vi "test - github 85 cannot write parameters into empty ini.vi"(8 "error in (no error)":errorcluster, 11 "TestCase in":refnum<class "csm-ini-variable-addon.lvclass">) -> (0 "error out":errorcluster, 3 "TestCase out":refnum<class "csm-ini-variable-addon.lvclass">)   [LabVIEW 2017, in "csm-ini-variable-addon.lvclass"]
uses:
  csm-ini-variable-addon.lvclass
  fd1f1403-f650-4147-a5d0-7fa8994ff20a.vi
  a890fef7-7f1d-42c9-b9db-12bb2b441289.vi
  25df91f5-a8e9-4b30-a15a-ad417606420d.vi
  4506128f-911b-4b09-9ad5-a28d51cf287f.vi
  fd1f1403-f650-4147-a5d0-7fa8994ff20a.vi/99de0c97-112a-4c86-9094-c187659127e1.vi
  <vilib>/Utility/error.llb/Clear Errors.vi
  a890fef7-7f1d-42c9-b9db-12bb2b441289.vi/99de0c97-112a-4c86-9094-c187659127e1.vi
  25df91f5-a8e9-4b30-a15a-ad417606420d.vi/99de0c97-112a-4c86-9094-c187659127e1.vi
  4506128f-911b-4b09-9ad5-a28d51cf287f.vi/99de0c97-112a-4c86-9094-c187659127e1.vi
  <vilib>/Utility/Data Type/Get Type Information.vi
  <userlib>/_NEVSTOP/Communicable State Machine(CSM)/addons/API-String-Arugments-Support/_Support/Data To SingleElementsArray_csm.vi
  <userlib>/_NEVSTOP/Communicable State Machine(CSM)/addons/API-String-Arugments-Support/_Support/Data To API String Arguments.vi
  INI-Static-Variable-Support/_Support/Parse Used Session and Name.vi
  INI-Static-Variable-Support/_Support/INI-FGV(lvlibp).vi
  INI-Static-Variable-Support/INI-Static-Variable-Support.lvlib
panel:
  # "Connector Pane"
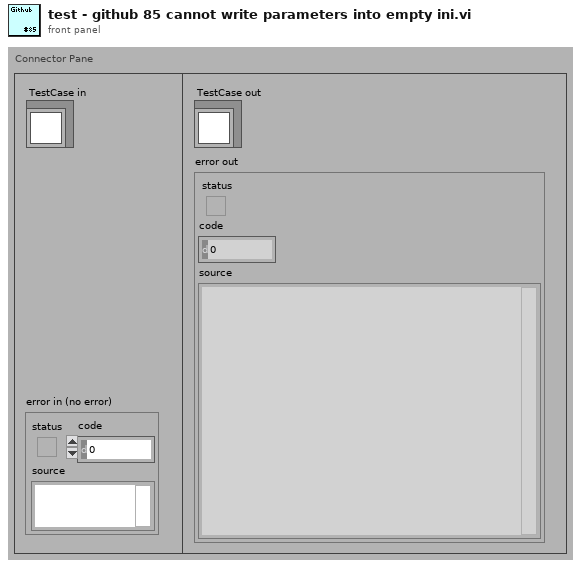
[diagram p1: front panel]
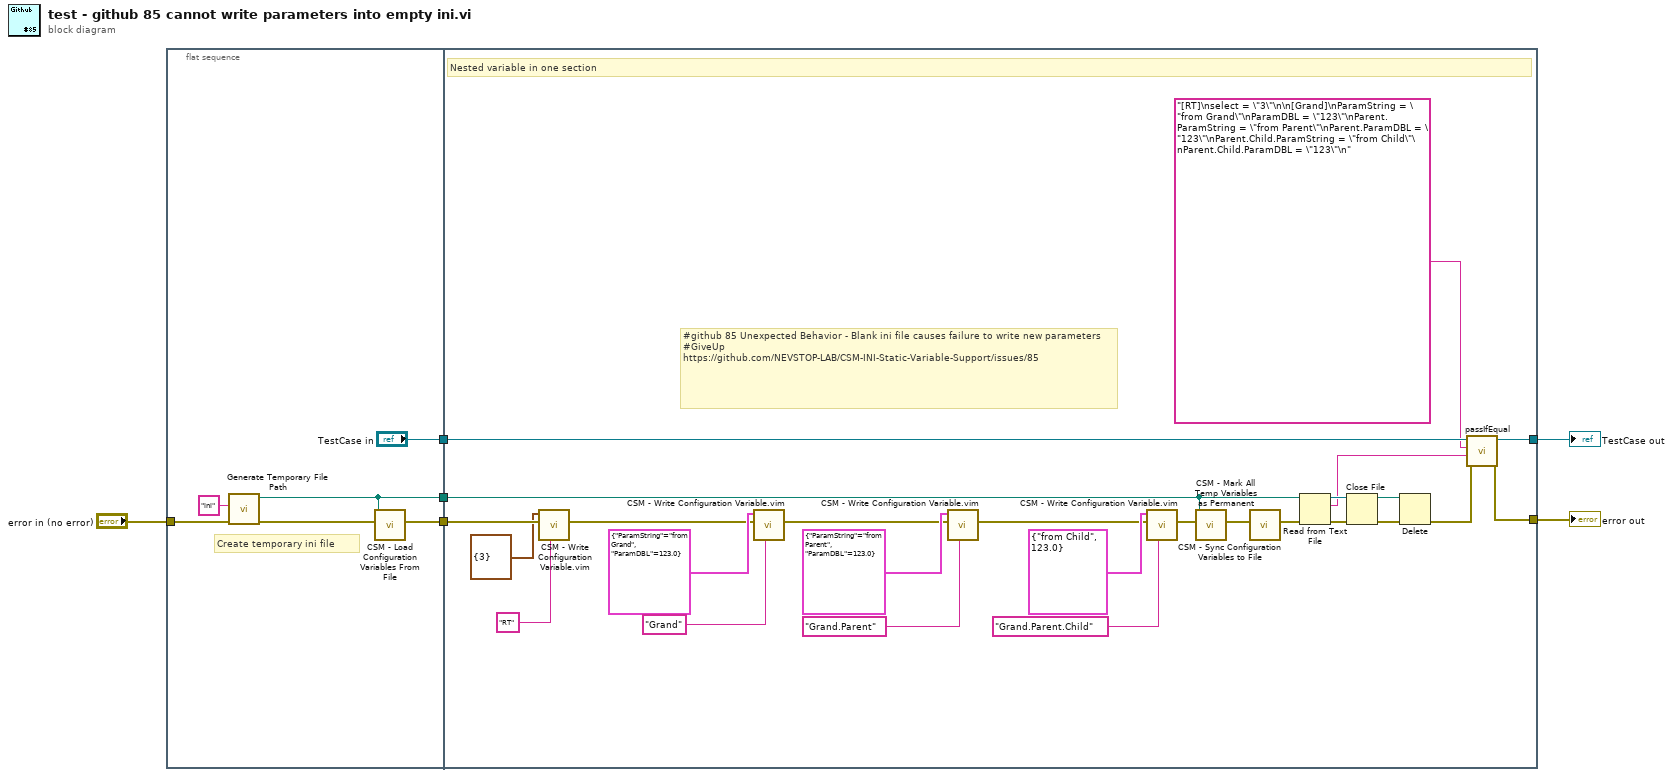
[diagram p0: block diagram]
diagram:
  n1 = flat-sequence {
    tunnel: "error in (no error)" -> [w11]
    tunnel: [w9] -> w5
    tunnel: ["TestCase in"] -> w4
    tunnel: [w7] -> w1
    tunnel: w5 -> [w35]
    tunnel: w4 -> [w34]
    tunnel: [w38] -> w3
    tunnel: [w37] -> w2
    tunnel: w1 -> [w36]
    frame #0 {
      # "Create temporary ini file"
      n2 = call <vilib>:"Generate Temporary File Path.vi"("error in (no error)"=w11, "Temporary File Extension (tmp)"="ini") -> ("error out"=w8:errorcluster, "Unique Temporary File Path"=w7:path)  [unwired: 8 in]
      n3 = call "CSM - Load Configuration Variables From File.vi"("error in (no error)"=w8, "Configuration Path"=w7) -> ("error out"=w9:errorcluster)  [unwired: 7 in]
    }
    frame #1 {
      # "#github 85 Unexpected Behavior - Blank ini file causes failure to write new parameters #GiveUp\nhttps://github.com/NEVSTOP-LAB/CSM-INI-Static-Variable-Support/issues/85"
      # "Nested variable in one section"
      n4 = call "CSM - Write Configuration Variable.vim"("Section Name (\"\" as Default)"="RT" ("Section Name(\"\" as Default)"), "error in (no error)"=w35, "Configuration"=cluster{"select":i32} {"select"=3}) -> ("error out"=w18:errorcluster)  [unwired: 5 in, 1 out]
      n5 = call "CSM - Write Configuration Variable.vim"("Section Name (\"\" as Default)"="Grand" ("Section Name(\"\" as Default)"), "error in (no error)"=w18, "Configuration"=cluster{"ParamString":string, "ParamDBL":dbl} {"ParamString"="from Grand", "ParamDBL"=123.0}) -> ("error out"=w29:errorcluster)  [unwired: 5 in, 1 out]
      n6 = call "CSM - Write Configuration Variable.vim"("Section Name (\"\" as Default)"="Grand.Parent" ("Section Name(\"\" as Default)"), "error in (no error)"=w29, "Configuration"=cluster{"ParamString":string, "ParamDBL":dbl} {"ParamString"="from Parent", "ParamDBL"=123.0}) -> ("error out"=w26:errorcluster)  [unwired: 5 in, 1 out]
      n7 = call "CSM - Write Configuration Variable.vim"("Section Name (\"\" as Default)"="Grand.Parent.Child" ("Section Name(\"\" as Default)"), "error in (no error)"=w26, "Configuration"=cluster{"ParamString":string, "ParamDBL":dbl} {"ParamString"="from Child", "ParamDBL"=123.0}) -> ("error out"=w25:errorcluster)  [unwired: 5 in, 1 out]
      n8 = call "CSM - Mark All Temp Variables as Permanent.vi"("error in (no error)"=w25, "Path (\"\" to Use Default File)"=w36) -> ("error out"=w24:errorcluster)  [unwired: 7 in]
      n9 = call "CSM - Sync Configuration Variables to File.vi"("error in (no error)"=w24) -> ("error out"=w23:errorcluster)  [unwired: 8 in]
      n10 = Read from Text File(file (use dialog)=w36, error in=w23) -> (refnum out=w22:refnum<file>, text=w14:string, error out=w21:errorcluster)  [unwired: 2 in, 1 out]
      n11 = Close File(refnum=w22, error in=w21) -> (path=w19:path, error out=w20:errorcluster)
      n12 = Delete(path (use dialog)=w19, error in=w20) -> (error out=w15:errorcluster)  [unwired: 3 in, 2 out]
      n13 = call-dynamic "passIfEqual.vi"("error in (no error)"=w15, "y"=w14, "x"="[RT]\nselect = \"3\"\n\n[Grand]\nParamString = \"from Grand\"\nParamDBL = \"123\"\nParent.ParamString = \"from Parent\"\nParent.ParamDBL = \"123\"\nParent.Child.ParamString = \"from Child\"\nParent.Child.ParamDBL = \"123\"\n" ("text"), "TestCase in"=w34) -> ("error out"=w37:errorcluster, "TestCase out"=w38:refnum<class "csm-ini-variable-addon.lvclass">)  [unwired: 6 in]
    }
  }
  "error out" <- w2
  "TestCase out" <- w3
